vi "LEDs整体图.vi"() -> ()   [LabVIEW 2014]
panel:
  in  "Light green":bool
  in  "Green":bool
  in  "Cyan":bool
  in  "Blue":bool
  in  "Yellow":bool
  in  "Red":bool
  in  "Record":bool
  in  "Purple":bool
  in  "Orange":bool
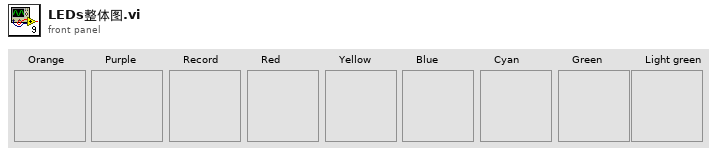
[diagram p1: front panel]
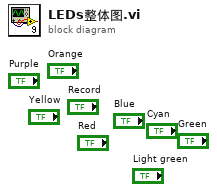
[diagram p0: block diagram]
diagram:
